vi "Method.vi"(4 "B":refnum<class "Abs_Boolean.lvclass">, 5 "A":refnum<class "Abs_Boolean.lvclass">) -> (1 "Result":refnum<class "Abs_Boolean.lvclass">)   [LabVIEW 2021, in "OR_Bool.lvclass"]
uses:
  OR_Bool.lvclass
  Abs_Types/Boolean/Abs_Boolean.lvclass
  C:/TSA/LV_Abstract/Source/Functions/Support/Function/Two Terminal/Boolean/AbsFunc_Two Term_Bool.lvclass
  C:/Program Files (x86)/National Instruments/LabVIEW 2021/vi.lib/TSA/Abstract Data Classes/Abs_Types/Boolean/Abs_Boolean.lvclass
  Support/Function/Two Terminal/Boolean/AbsFunc_Two Term_Bool.lvclass/AbsFunc_Two Term_Bool.ctl
  Support/Function/Two Terminal/Boolean/Properties/Write Bool A.vi
  Support/Function/Two Terminal/Boolean/Properties/Write Bool B.vi
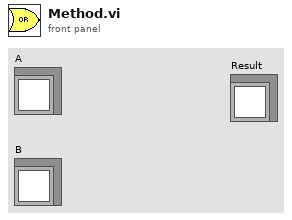
[diagram p1: front panel]
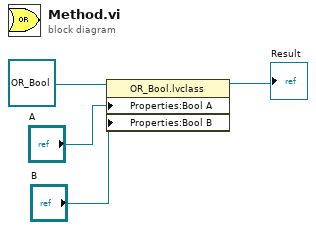
[diagram p0: block diagram]
diagram:
  n1 = property class="OR_Bool.lvclass"(reference=refnum<class "OR_Bool.lvclass"> refnum ("OR_Bool.lvclass"), "Properties:Bool A"="A", "Properties:Bool B"="B") -> (reference out=→"Result":refnum<class "OR_Bool.lvclass">)  [unwired: 1 in, 1 out]
